vi "Graph1.vi"() -> ()   [LabVIEW 2019]
uses:
  Supported.llb/Global-1.vi
panel:
  out "Lower":cluster{"x":dbl[], "y":dbl[]}
  out "Upper":cluster{"x":dbl[], "z":dbl[]}
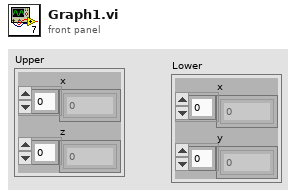
[diagram p1: front panel]
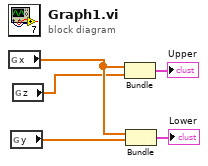
[diagram p0: block diagram]
diagram:
  n1 = global read "Global-1.vi" "x"() -> (w5:dbl[])
  n2 = global read "Global-1.vi" "y"() -> (w3:dbl[])
  n3 = global read "Global-1.vi" "z"() -> (w4:dbl[])
  n4 = Bundle("x"=w5, "z"=w4) -> (→"Upper":cluster{"x":dbl[], "z":dbl[]})  [unwired: 1 in]
  n5 = Bundle("x"=w5, "y"=w3) -> (→"Lower":cluster{"x":dbl[], "y":dbl[]})  [unwired: 1 in]
